vi "Map to Directions.vi"(8 "error in (no error)":errorcluster, 10 "Direction Heading":T1, 11 "Grassfire Algorithm in":refnum<class "Grassfire Algorithm.lvclass">) -> (0 "error out":errorcluster, 2 "Directions":T1[](array[typedef]), 3 "Grassfire Algorithm out":refnum<class "Grassfire Algorithm.lvclass">)   [LabVIEW 2019, in "Grassfire Algorithm.lvclass"]
uses:
  Grassfire Algorithm.lvclass
  Direction--enum.ctl
  Index Column Row--cluster.ctl
  Grassfire Algorithm.lvclass/Grassfire Algorithm.ctl
  Solution--picture ring.ctl
  <userlib>/_OpenG.lib/array/array.llb/Sort 1D Array (DBL)__ogtk.vi
  <userlib>/_OpenG.lib/array/array.llb/Reorder 1D Array2 (I16)__ogtk.vi
panel:
  out "i":i32
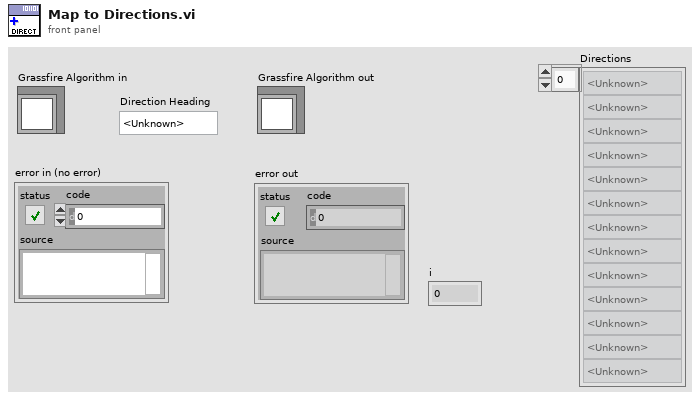
[diagram p1: front panel]
types:
  T1 = typedef "Grassfire Algorithm.lvclass/Direction--enum.ctl" = enum16{"<Unknown>", "Right", "Down", "Left", "Up"}
  T2 = typedef "Grassfire Algorithm.lvclass/Index Column Row--cluster.ctl" = cluster{"Row":i32, "Column":i32}
  T3 = typedef "Grassfire Algorithm.lvclass/Solution Grid Cell Private--cluster.ctl" = cluster{"Picture":T4, "Value":dbl}
  T4 = typedef "Grassfire Algorithm.lvclass/Solution--picture ring.ctl" = i64
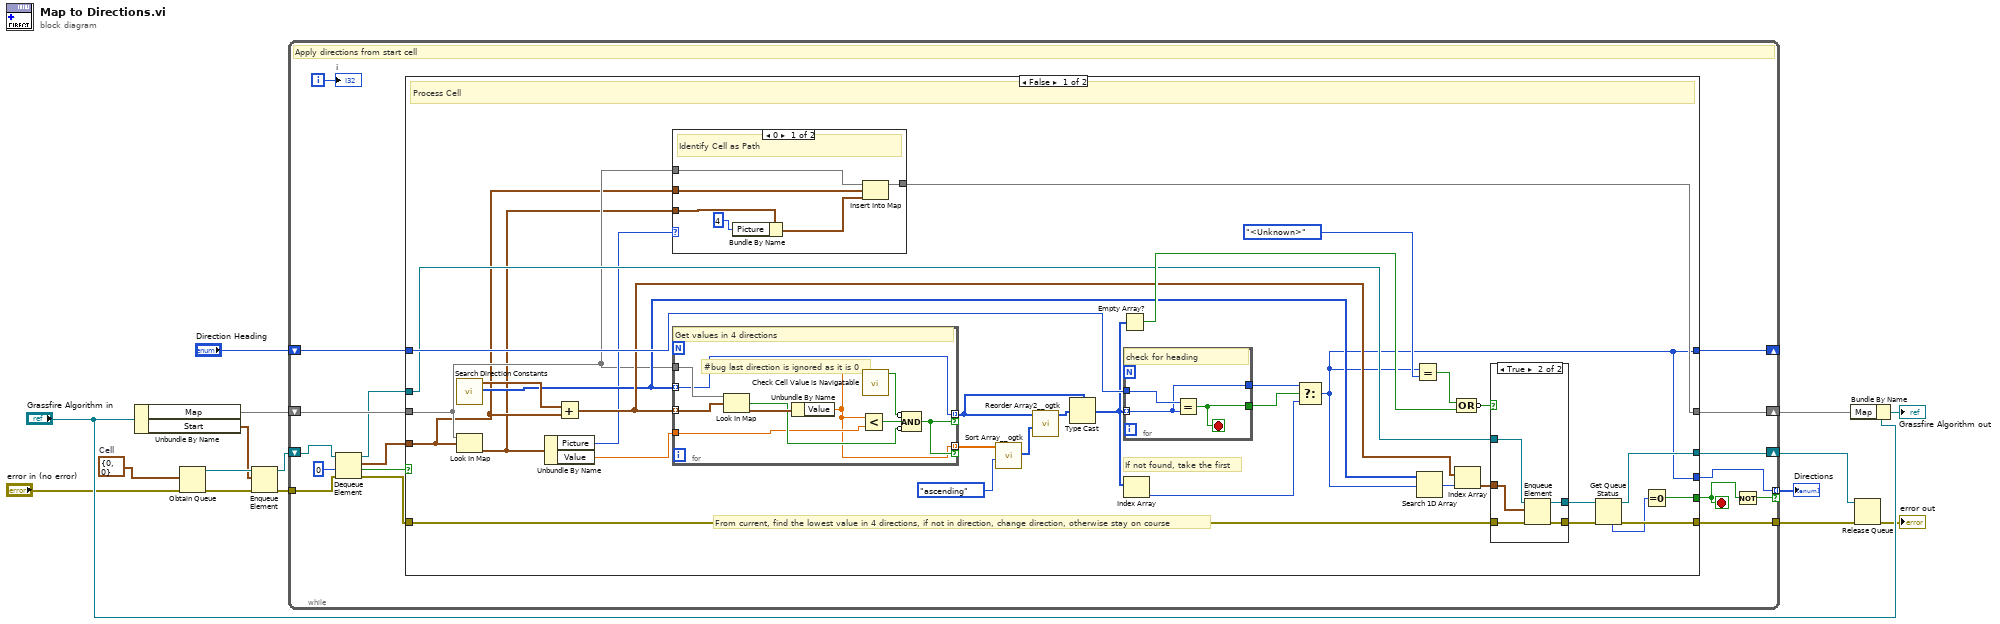
[diagram p0: block diagram]
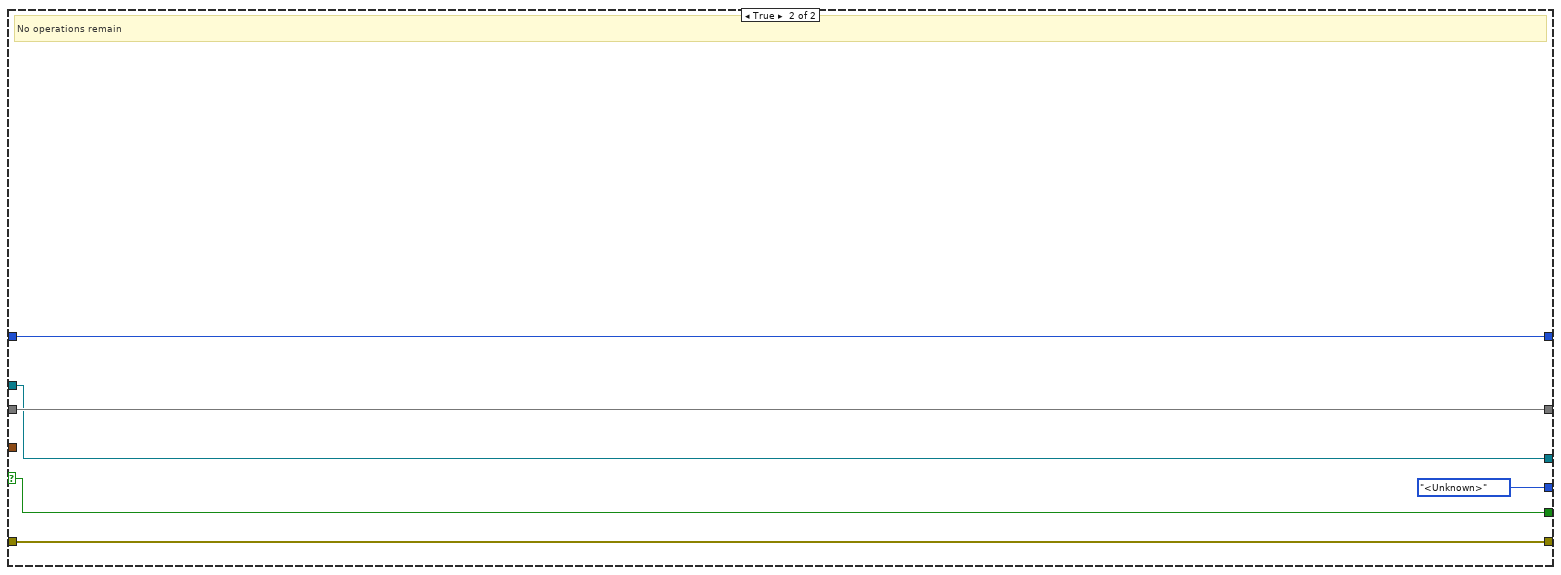
[diagram p4: hidden frame]
diagram:
  w4 = T2 {"Row"=0, "Column"=0}  # Cell
  n1 = Unbundle By Name("Grassfire Algorithm in") -> ("Map"=w15:map{T2, T3}, "Start"=w3:T2)
  n2 = Obtain Queue(element data type=w4, error in (no error)="error in (no error)") -> (queue out=w13:refnum<queue>, error out=w11:errorcluster)  [unwired: 3 in, 1 out]
  n3 = Enqueue Element(queue=w13, element=w3, error in (no error)=w11) -> (queue out=w12:refnum<queue>, error out=w10:errorcluster)  [unwired: 1 in, 1 out]
  n4 = while {
    shift-right: [w32] -> w16
    shift-left: w15 -> [w33]
    shift-right: [w22] -> w14
    shift-left: w12 -> [w28]
    tunnel: w10 -> [w25]
    tunnel: [w23] -> w9
    shift-right: [w21] -> _
    shift-left: "Direction Heading" -> [w20]
    tunnel: [w19] -> w1 mode=indexing if=w18
    i -> [w31]
    stop <- w17 stop-if-true
    # "Apply directions from start cell"
    n5 = Dequeue Element(queue=w28, timeout in ms (-1)=0, error in (no error)=w25) -> (queue out=w26:refnum<queue>, element=w27:T2, timed out?=w29:bool, error out=w24:errorcluster)
    n6 = case shown="False" w29 {
      selector: w29 -> [_ w97]
      tunnel: w33 -> [w42 w100]
      tunnel: [w41 w100] -> w32
      tunnel: w27 -> [w40 _]
      tunnel: w26 -> [w52 w99]
      tunnel: [w67 w99] -> w22
      tunnel: w24 -> [w51 w98]
      tunnel: [w66 w98] -> w23
      tunnel: [w65 w97] -> w17
      tunnel: [w34 w96] -> w21
      tunnel: w20 -> [w58 w96]
      tunnel: [w34 Direction--enum."<Unknown>" ("Direction Heading")] -> w19
      frame False {
        # "If not found, take the first"
        # "From current, find the lowest value in 4 directions, if not in direction, change direction, otherwise stay on course"
        # "Process Cell"
        n7 = call "Search Direction Constants.vi"() -> ("Search Directions"=w45:T1[], "Search Direction Cells"=w46:T2[])  [unwired: 10 in]
        n8 = Look In Map(map=w42, key=w40) -> (value=w39:T3)  [unwired: 1 in, 1 out]
        n9 = Unbundle By Name(w39) -> ("Picture"=w43:T4, "Value"=w44:dbl)
        n10 = Add(x=w46, y=w40) -> (x+y=w54:T2[])
        n11 = case shown="0" w43 {
          tunnel: [w73 w74] -> w41
          tunnel: w42 -> [w72 w74]
          tunnel: w40 -> [w71 _]
          tunnel: w39 -> [w70 _]
          frame 0 {
            # "Identify Cell as Path"
            n12 = Bundle By Name(cluster=w70, "Picture"=T4 4) -> (w69:T3)
            n13 = Insert Into Map(map in=w72, key=w71, value=w69) -> (map out=w73:map{T2, T3})  [unwired: 2 out]
          }
          frame Default {
          }
        }
        n14 = for {
          tunnel: w42 -> [w94]
          tunnel: w54 -> [w93] mode=indexing
          tunnel: [w86] -> w63 mode=indexing if=w89
          tunnel: [w91] -> w59 mode=indexing if=w89
          tunnel: w45 -> [w91] mode=indexing
          tunnel: w44 -> [w87]
          # "#bug last direction is ignored as it is 0"
          # "Get values in 4 directions"
          n15 = Look In Map(map=w94, key=w93) -> (key not found?=w90:bool, value=w92:T3)  [unwired: 1 in]
          n16 = Unbundle By Name(w92) -> ("Value"=w86:dbl)
          n17 = Less?(x=w86, y=w87) -> (x < y?=w88:bool)
          n18 = call "Check Cell Value is Navigatable.vi"("Value"=w86) -> ("Invalid Cell?"=w85:bool)  [unwired: 10 in]
          n19 = Compound Arithmetic op=AND(invert w85, w88, invert w90) -> (w89:bool)
        }
        n20 = call-poly <userlib>:"Sort Array__ogtk.vi"("Order"=enum16{"ascending", "descending"}."ascending", "Array in"=w63) -> ("Sorted Pointers"=w61:i32[])  [unwired: 8 in, 1 out]
        n21 = call-poly <userlib>:"Reorder Array2__ogtk.vi"("indices"=w61, "array"=w59) -> ("reordered array"=w60:i16[])  [unwired: 9 in]
        n22 = Type Cast(type=w59, x=w60) -> (*(type *) &x=w37:T1[])
        n23 = Empty Array?(array=w37) -> (empty?=w55:bool)
        n24 = for {
          tunnel: w37 -> [w83] mode=indexing
          tunnel: w58 -> [w84]
          tunnel: [w83] -> w36
          tunnel: [w82] -> w38
          stop <- w82 stop-if-true
          # "check for heading"
          n25 = Equal?(x=w84, y=w83) -> (x = y?=w82:bool)
        }
        n26 = Index Array(array=w37) -> (element=w35:T1)  [unwired: 1 in]
        n27 = Select(t=w36, s=w38, f=w35) -> (s? t:f=w34:T1)
        n28 = Equal?(x=w34, y=Direction--enum."<Unknown>") -> (x = y?=w56:bool)
        n29 = Search 1D Array(1D array=w45, element=w34) -> (index of element=w53:i32)  [unwired: 1 in]
        n30 = Index Array(array=w54, index=w53) -> (element=w48:T2)
        n31 = Compound Arithmetic op=OR(w56, w55) -> (invert w47:bool)
        n32 = case shown="True" w47 {
          tunnel: w52 -> [w76 w81]
          tunnel: w51 -> [w75 w80]
          tunnel: [w76 w79] -> w50
          tunnel: [w75 w78] -> w49
          tunnel: w48 -> [_ w77]
          frame False {
          }
          frame True {
            n33 = Enqueue Element(queue=w81, element=w77, error in (no error)=w80) -> (queue out=w79:refnum<queue>, error out=w78:errorcluster)  [unwired: 1 in, 1 out]
          }
        }
        n34 = Get Queue Status(queue=w50, error in (no error)=w49) -> (queue out=w67:refnum<queue>, error out=w66:errorcluster, # elements in queue=w64:i32)  [unwired: 1 in, 5 out]
        n35 = Equal To 0?(x=w64) -> (x = 0?=w65:bool)
      }
      frame True {
        # "No operations remain"
      }
    }
    n36 = Not(x=w17) -> (.not. x?=w18:bool)
    "i" <- w31
  }
  "Directions" <- w1
  n37 = Bundle By Name(cluster="Grassfire Algorithm in", "Map"=w16) -> (→"Grassfire Algorithm out":refnum<class "Grassfire Algorithm.lvclass">)
  n38 = Release Queue(queue=w14, error in (no error)=w9) -> (error out=→"error out":errorcluster)  [unwired: 1 in, 2 out]
